vi "Unflatten Value.vi"(8 "error in (no error)":errorcluster, 10 "Value":string, 11 "Boolean in":refnum<class "I32 1D.lvclass">) -> (0 "error out":errorcluster, 3 "Boolean out":refnum<class "I32 1D.lvclass">)   [LabVIEW 2020, in "I32 1D.lvclass"]
uses:
  <vilib>/gpm_packages/@cs/data-type-serializer/source/I32 1D/I32 1D.lvclass
  <vilib>/gpm_packages/@cs/data-type-serializer/source/I32 1D/I32 1D.lvclass/I32 1D.ctl
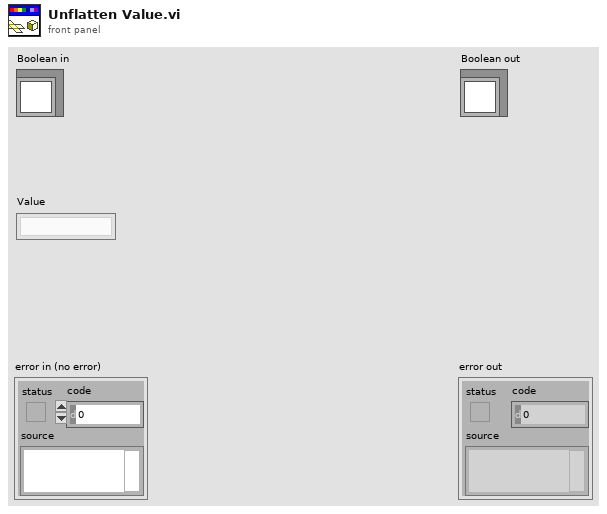
[diagram p1: front panel]
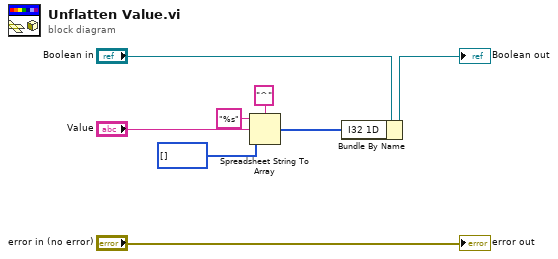
[diagram p0: block diagram]
diagram:
  n1 = Spreadsheet String To Array(delimiter (Tab)="^", format string="%s", spreadsheet string="Value", array type (2D Dbl)=i32[] [] ("Double 1D")) -> (array=w1:i32[])
  n2 = Bundle By Name(cluster="Boolean in", "I32 1D"=w1) -> (→"Boolean out":refnum<class "I32 1D.lvclass">)
  "error out" <- "error in (no error)"
